vi "Update Shutter.vi"(8 "error in (no error)":errorcluster caption="entrée d'erreur (pas d'erreur)", 9 "Shutter":dbl, 10 "IMAQdx Session in":T1, 11 "Acq Cam Basler en entrée":refnum<class "Acq Cam Basler.lvclass">) -> (0 "error out":errorcluster caption="sortie d'erreur", 2 "IMAQdx Session out":T1, 3 "Acq Cam Basler en sortie":refnum<class "Acq Cam Basler.lvclass">)   [LabVIEW 2023, in "Acq Cam Basler.lvclass"]
uses:
  Acq Cam Basler.lvclass
  <vilib>/userDefined/High Color/IMAQdx.ctl
  Acq Cam Basler.lvclass/Acq Cam Basler.ctl
  <vilib>/Utility/error.llb/Error Cluster From Error Code.vi
  <vilib>/ErrorRing/Error Ring.xnode
  <resource>/objmgr/imaqdx.rc
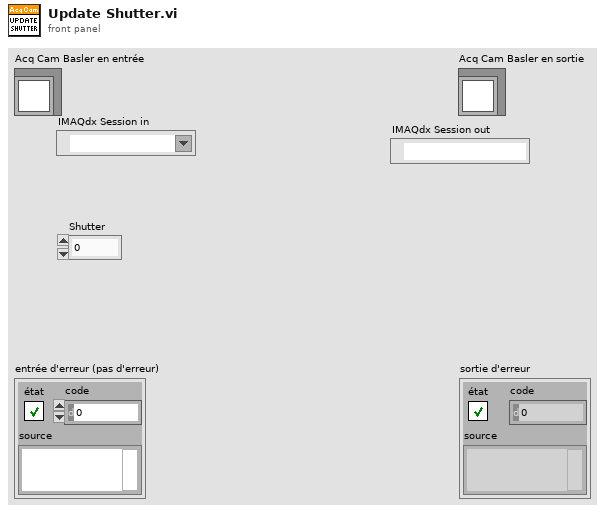
[diagram p1: front panel]
types:
  T1 = typedef "IMAQdx.ctl" = refnum<k21>
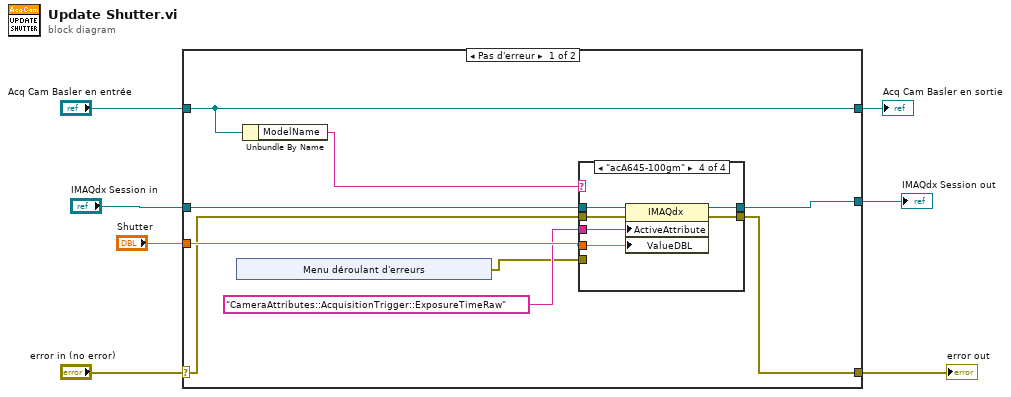
[diagram p0: block diagram]
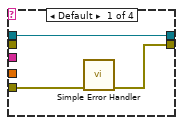
[diagram p2: hidden frame]
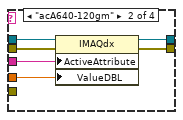
[diagram p3: hidden frame]
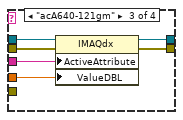
[diagram p4: hidden frame]
diagram:
  n1 = case shown="Pas d'erreur" "error in (no error)" {
    selector: "error in (no error)" -> [w15 w45]
    tunnel: [w14 w45] -> w6
    tunnel: [w10 w44] -> w4
    tunnel: "Acq Cam Basler en entrée" -> [w10 w44]
    tunnel: "Shutter" -> [w16 _]
    tunnel: [w13 w43] -> w2
    tunnel: "IMAQdx Session in" -> [w12 w43]
    frame No Error {
      n2 = xnode "Menu déroulant d'erreurs"() -> ("sortie d'erreur"=w8:errorcluster)
      n3 = Unbundle By Name(w10) -> ("ModelName"=w9:string)
      n4 = case shown="\"acA645-100gm\"" w9 {
        tunnel: w16 -> [_ w30 w36 w42]
        tunnel: w15 -> [_ w29 w35 w41]
        tunnel: [w23 w28 w34 w40] -> w14
        tunnel: [w22 w27 w33 w39] -> w13
        tunnel: w12 -> [w22 w26 w32 w38]
        tunnel: "CameraAttributes::AcquisitionTrigger::ExposureTimeRaw" ("ActiveAttribute") -> [_ w25 w31 w37]
        tunnel: w8 -> [w24 _ _ _]
        frame Default {
          n5 = call <vilib>:"Simple Error Handler.vi"("error in (no error)"=w24) -> ("error out"=w23:errorcluster)  [unwired: 4 in, 4 out]
        }
        frame "acA640-120gm" {
          n6 = property class="IMAQdx"(reference=w26, error in=w29, "ActiveAttribute"=w25, "ValueDBL"=w30) -> (reference out=w27:T1, error out=w28:errorcluster)
        }
        frame "acA640-121gm" {
          n7 = property class="IMAQdx"(reference=w32, error in=w35, "ActiveAttribute"=w31, "ValueDBL"=w36) -> (reference out=w33:T1, error out=w34:errorcluster)
        }
        frame "acA645-100gm" {
          n8 = property class="IMAQdx"(reference=w38, error in=w41, "ActiveAttribute"=w37, "ValueDBL"=w42) -> (reference out=w39:T1, error out=w40:errorcluster)
        }
      }
    }
    frame Error {
    }
  }
  "error out" <- w6
  "Acq Cam Basler en sortie" <- w4
  "IMAQdx Session out" <- w2
